vi "InitWithTopDocument.vi"(8 "error in":errorcluster, 11 "Device  In":T2) -> (0 "error out":errorcluster, 2 "Comm":T1, 3 "Device Out":T2)   [LabVIEW 2019]
uses:
  <userlib>/IoT Devices/_subVIs/HTTPComm.ctl
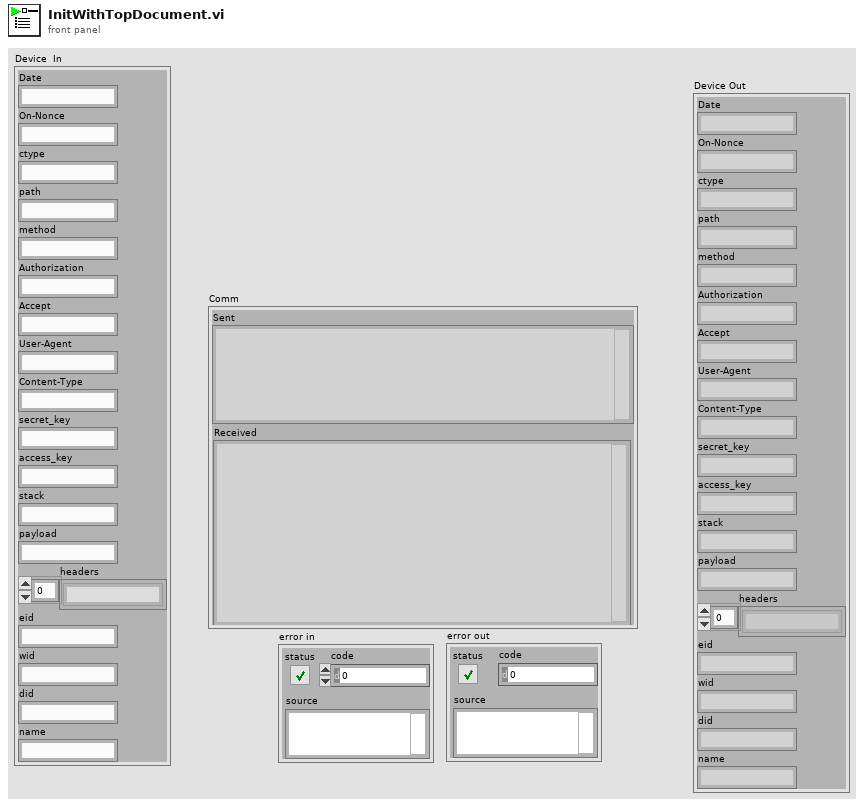
[diagram p1: front panel]
types:
  T1 = typedef "HTTPComm.ctl" = cluster{"url":string, "sent headers":string, "sent body":string, "headers":string, "body":string, "Sent":string, "Received":string}
  T2 = cluster{"Date":string, "On-Nonce":string, "ctype":string, "path":string, "method":string, "Authorization":string, "Accept":string, "User-Agent":string, "Content-Type":string, "secret_key":string, "access_key":string, "stack":string, "payload":string, "headers":string[], "eid":string, "wid":string, "did":string, "name":string}
  T3 = cluster{"items":cluster{"resourceType":string, "id":string, "name":string, "defaultWorkspace":cluster{"id":string}}[]}
  T4 = cluster{"resourceType":string, "id":string, "name":string, "defaultWorkspace":cluster{"id":string}}[]
  T5 = cluster{"resourceType":string, "id":string, "name":string, "defaultWorkspace":cluster{"id":string}}
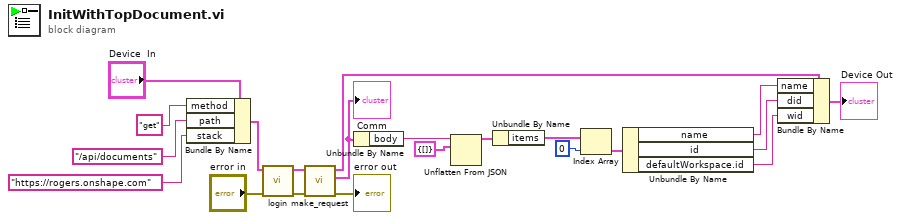
[diagram p0: block diagram]
diagram:
  n1 = Bundle By Name(cluster="Device  In", "method"="get" ("Method"), "path"="/api/documents" ("payload"), "stack"="https://rogers.onshape.com" ("stacks")) -> (w10:T2)
  n2 = call <userlib>:"login.vi"("error in"="error in", "Device In"=w10) -> ("error out"=w11:errorcluster, "Device Out"=w9:T2)  [unwired: 8 in]
  n3 = call <userlib>:"make_request.vi"("Error in"=w11, "Device In"=w9) -> ("error out"=→"error out":errorcluster, "Comm"=w16:T1, "Device Out"=w5:T2)  [unwired: 7 in]
  "Comm" <- w16
  n4 = Unbundle By Name(w16) -> ("body"=w15:string)
  n5 = Unflatten From JSON(JSON string=w15, type and defaults=T3 {"items"=[]}) -> (value=w13:T3)  [unwired: 5 in, 1 out]
  n6 = Unbundle By Name(w13) -> ("items"=w8:T4)
  n7 = Index Array(array=w8, index=0) -> (element=w6:T5)
  n8 = Unbundle By Name(w6) -> ("name"=w4:string, "id"=w3:string, "defaultWorkspace.id"=w2:string)
  n9 = Bundle By Name(cluster=w5, "name"=w4, "did"=w3, "wid"=w2) -> (→"Device Out":T2)
